vi "Initialize Waveforms V3.vi"(0 "Image Acquisition Parameters":T2={"Scan Type"=enum."Sample Scanning", "Scan Mode"=enum."XY", "Fast Axis Frequency (Hz)"=100.0, "Image Format"=128, "Line Accumulations"=1, "Frames Per Capture"=1, "Frames Accumulations"=1, "Image Dimension (um)"=[], "Number of Z Steps"=1, "Z Steps Size (um)"=1.0, "Pixel Size (nm)"=[]} {"Z Steps Size (um)" min=0.0; "Number of Z Steps" min=1; "Frames Accumulations" min=1; "Frames Per Capture" min=1; "Line Accumulations" min=1; "Image Format" items=["64 x 64"=64, "128 x 128"=128, "256 x 256"=256, "512 x 512"=512, "1024 x 1024"=1024, "2048 x 2048"=2048]}, 11 "Galvo Scale Factor":dbl=0.5 format="%#_13g") -> (4 "Waveform Data":T1)   [LabVIEW 2016]
uses:
  Type Defs/Image Acquisition Parameters.ctl
  Waveform Data.ctl
panel:
  in  "Waveform Data":T1
  out "Fast":cluster{dbl[], dbl[]}(graph)
  in  "Number Data of Points":i32=5000
  out "np":i32=5520
  out "total # lines":i32=296
  out "Slow":cluster{"t":dbl[], "L":dbl[]}(graph)
  out "% active scan":dbl=92.7536231884058
  out "dt":dbl=6.169792694965449e-06
  out "slow freq (Hz)":dbl=29.36231884057971
  out "T":dbl=0.03405725567620928
  out "t0":dbl=0.032823297137216184
  out "max dh/dt (V/s)":dbl=-1980.1192841578468
  out "constraint":dbl=7537.739130434783
  out "dh":dbl=0.07812500000000001
  out "k":dbl=7463.978793397228
  out "delta t (s)":dbl=0.0024679170779861796
  out "scan slope":dbl=31.656250000000004
  out "t image (s)":dbl=0.0315893385982231
  out "# lines flyback":i16=40
  in  "beta":dbl=0.0001 format="%0.2p"
  # "Copyright (C) 2010 Travis Gould\nCopyright (C) 2020 Edward S Allgeyer\n\nRedistribution and use in source and binary forms, with or without\nmodification, are permitted provided that the following conditions\nare met:\n\n1. Redistributions of source code must retain the above copyright\n   notice, this list of conditions and the following disclaimer.\n\n2. Redistributions in binary form must reproduce the above copyright\n   notice, this list of conditions and the following disclaimer in\n   the documentation and/or other materials provided with the\n   distribution.\n\n3. Neither the name of the copyright holder nor the names of its\n   contributors may be used to endorse or promote products derived\n   from this software without specific prior written permission.\n\nTHIS SOFTWARE IS PROVIDED BY THE COPYRIGHT HOLDERS AND CONTRIBUTORS\n\"AS IS\" AND ANY EXPRESS OR IMPLIED WARRANTIES, INCLUDING, BUT NOT\nLIMITED TO, THE IMPLIED WARRANTIES OF MERCHANTABILITY AND FITNESS\nFOR A PARTICULAR PURPOSE ARE DISCLAIMED. IN NO EVENT SHALL THE\nCOPYRIGHT HOLDER OR CONTRIBUTORS BE LIABLE FOR ANY DIRECT, INDIRECT,\nINCIDENTAL, SPECIAL, EXEMPLARY, OR CONSEQUENTIAL DAMAGES (INCLUDING,\nBUT NOT LIMITED TO, PROCUREMENT OF SUBSTITUTE GOODS OR SERVICES;\nLOSS OF USE, DATA, OR PROFITS; OR BUSINESS INTERRUPTION) HOWEVER\nCAUSED AND ON ANY THEORY OF LIABILITY, WHETHER IN CONTRACT, STRICT\nLIABILITY, OR TORT (INCLUDING NEGLIGENCE OR OTHERWISE) ARISING IN\nANY WAY OUT OF THE USE OF THIS SOFTWARE, EVEN IF ADVISED OF THE\nPOSSIBILITY OF SUCH DAMAGE."
  # "XY"
  # "Z"
  # "Length"
  # "Height"
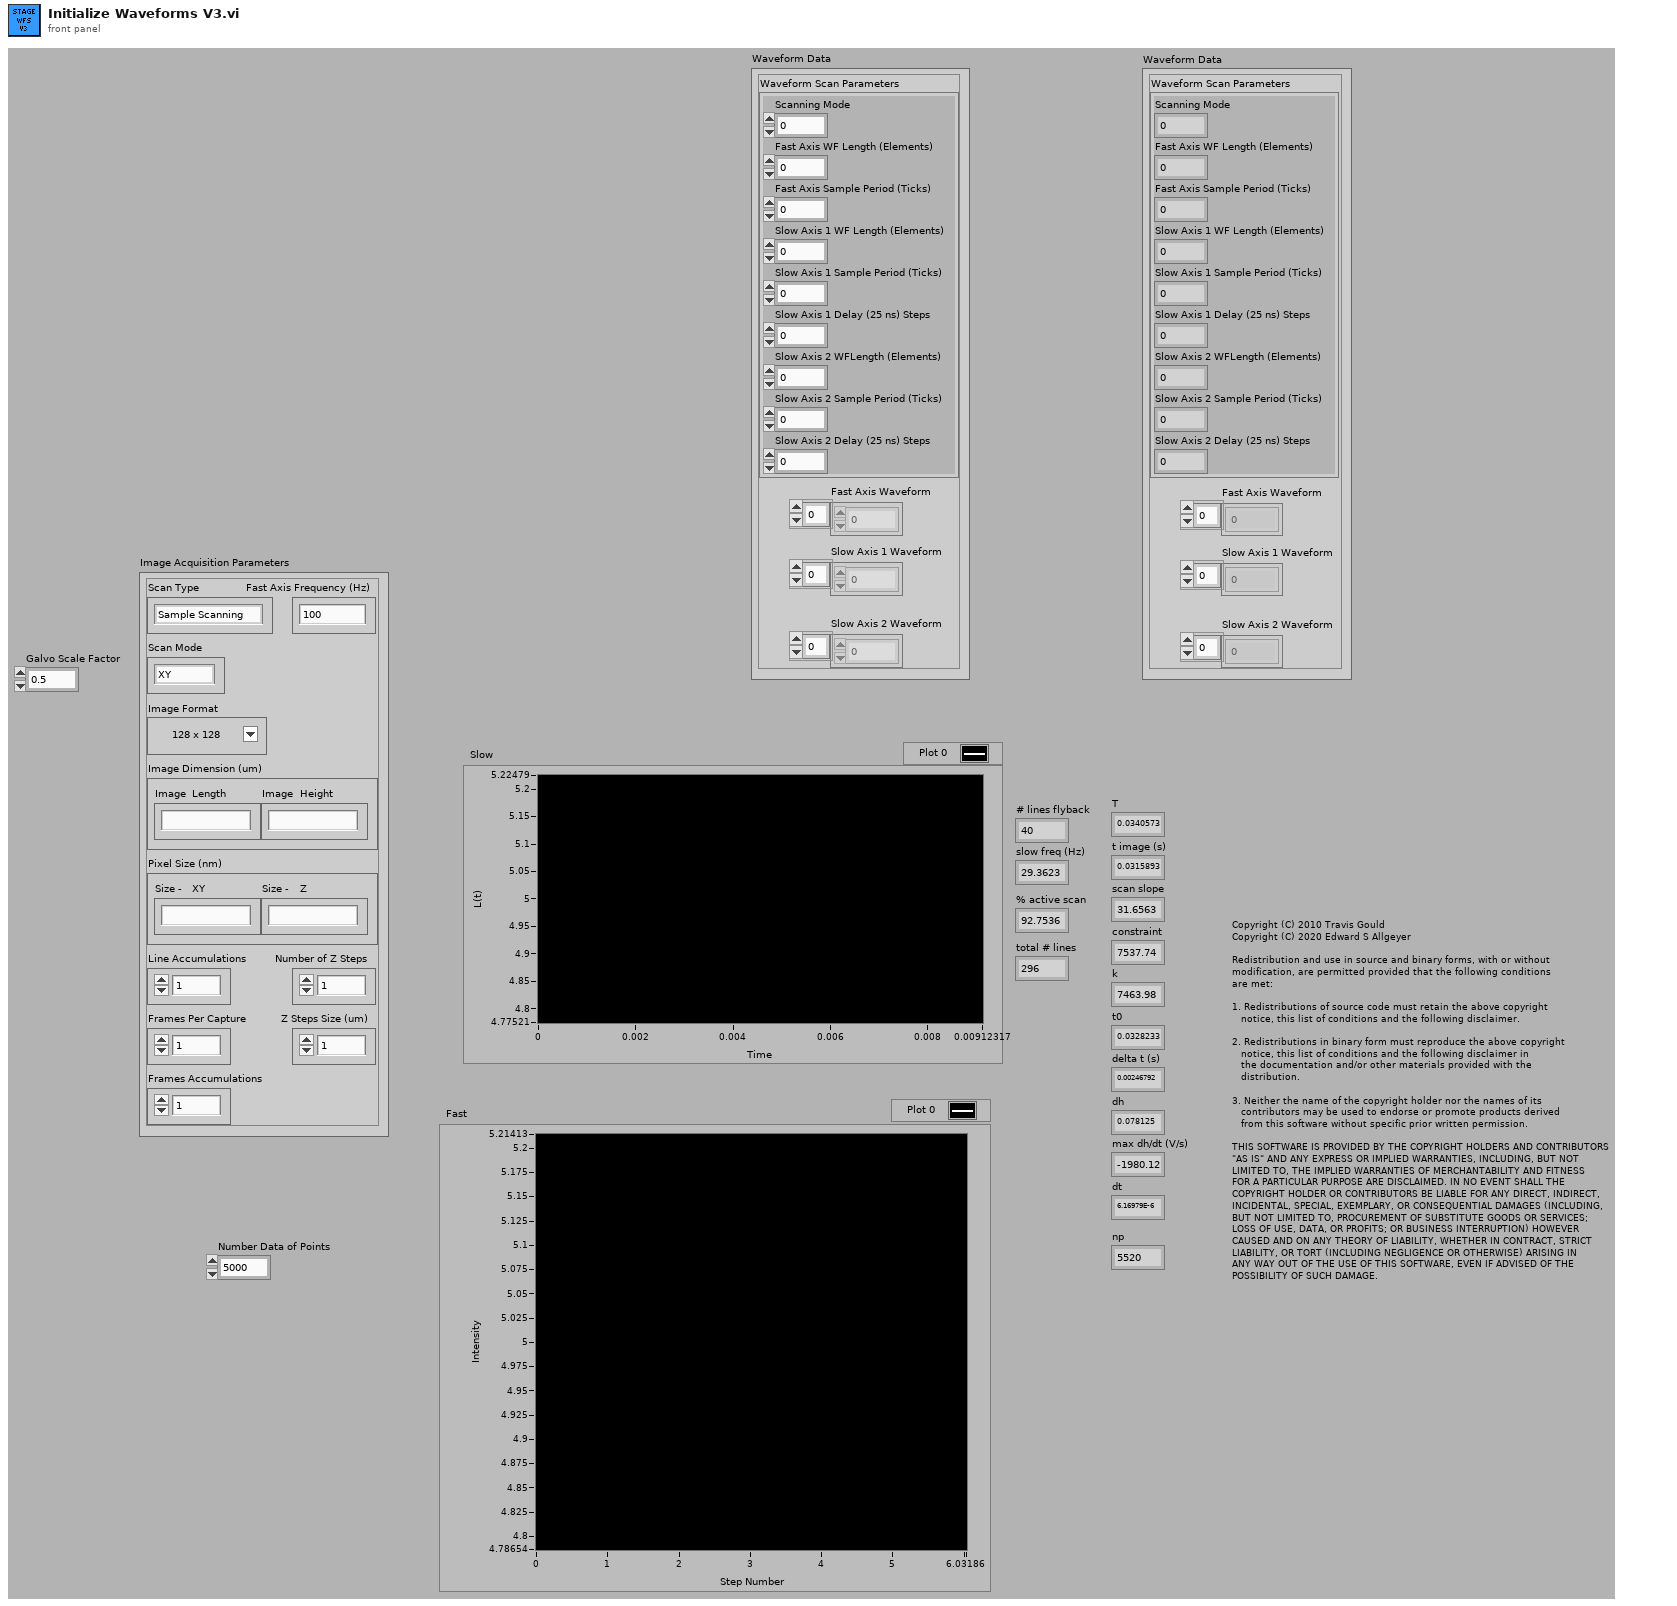
[diagram p1: front panel]
types:
  T1 = typedef "Waveform Data.ctl" = cluster{"Waveform Scan Parameters":cluster{"Scanning Mode":u8, "Fast Axis WF Length (Elements)":i32, "Fast Axis Sample Period (Ticks)":u32, "Slow Axis 1 WF Length (Elements)":i32, "Slow Axis 1 Sample Period (Ticks)":u32, "Slow Axis 1 Delay (25 ns) Steps":i32, "Slow Axis 2 WFLength (Elements)":i32, "Slow Axis 2 Sample Period (Ticks)":u32, "Slow Axis 2 Delay (25 ns) Steps":i32}, "Fast Axis Waveform":dbl[], "Slow Axis 1 Waveform":dbl[], "Slow Axis 2 Waveform":dbl[]}
  T2 = typedef "Image Acquisition Parameters.ctl" = cluster{"Scan Type":enum16{"Sample Scanning", "Beam Scanning"}, "Scan Mode":enum16{"XY", "XZ", "YZ", "XYZ"}, "Fast Axis Frequency (Hz)":dbl, "Image Format":u16, "Line Accumulations":u16, "Frames Per Capture":u16, "Frames Accumulations":u16, "Image Dimension (um)":dbl[], "Number of Z Steps":u8, "Z Steps Size (um)":dbl, "Pixel Size (nm)":dbl[]}
  T3 = cluster{"Scanning Mode":u8, "Fast Axis WF Length (Elements)":i32, "Fast Axis Sample Period (Ticks)":u32, "Slow Axis 1 WF Length (Elements)":i32, "Slow Axis 1 Sample Period (Ticks)":u32, "Slow Axis 1 Delay (25 ns) Steps":i32, "Slow Axis 2 WFLength (Elements)":i32, "Slow Axis 2 Sample Period (Ticks)":u32, "Slow Axis 2 Delay (25 ns) Steps":i32}
  T4 = typedef "Scan Parameters.ctl" = cluster{"Fast_Ax_Amp_V":dbl, "Fast_Ax_Off_V":dbl, "Slow_Ax_Amp_V":dbl, "Slow_Ax_Off_V ":dbl, "Slow_Ax_Max_V_VperS":dbl, "Slow_Ax1_Del25ns":i32, "Slow_Ax2_Del25ns":i32, "Stage_X_Off_V":dbl, "Stage_Y_Off_V":dbl, "Stage_Z_Off_V":dbl, "Galvo1_Off_V":dbl, "Galvo2_Off_V":dbl, "Last_Scan_Mode":enum16{"XY", "XZ", "YZ", "XYZ"}, "Current_Scan_Mode":enum16{"XY", "XZ", "YZ", "XYZ"}, "Fly_Back_Lines":u16, "Linear_Ramp_End":u32, "Z_Step_I16":i16, "Z_Start_I16":i16, "Laser_States _U32":u32, "590_Voltage_I16":i16, "775_AOM_Volt_I16":i16, "Blanking OFF":bool, "Unused_Axis_I16":i16}
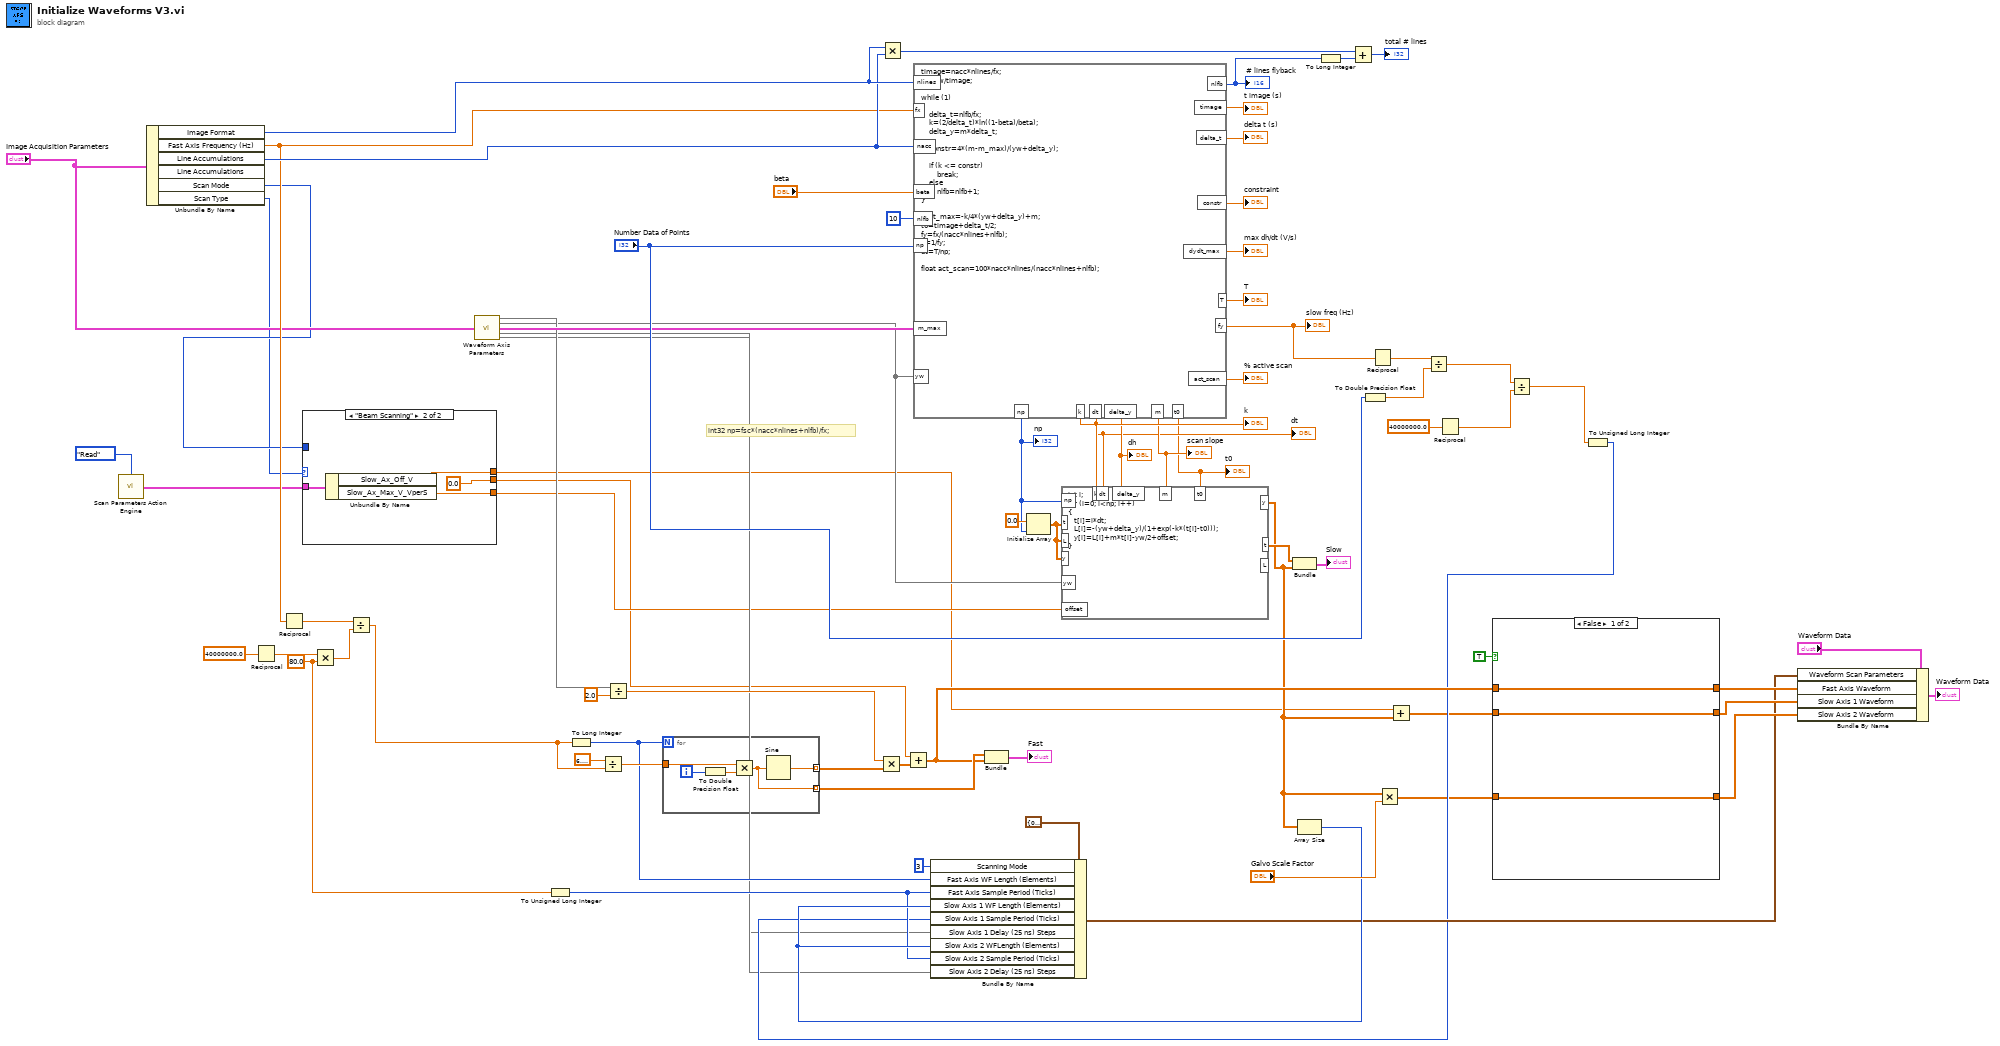
[diagram p0: block diagram]
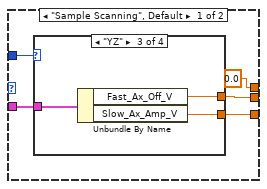
[diagram p2: hidden frame]
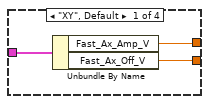
[diagram p3: hidden frame]
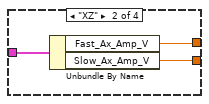
[diagram p4: hidden frame]
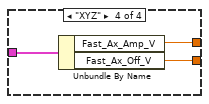
[diagram p5: hidden frame]
diagram:
  w33 = 80.0 ("y")
  # "int32 np=fsc*(nacc*nlines+nlfb)/fx;"
  n1 = call "Scan Parameters Action Engine.vi"("Action"=enum16{"Read", "Write"}."Read") -> ("Scan Parameters OUT"=w9:T4)  [unwired: 14 in]
  n2 = Unbundle By Name("Image Acquisition Parameters") -> ("Image Format"=w56:u16, "Fast Axis Frequency (Hz)"=w45:dbl, "Line Accumulations"=w55:u16, "Scan Mode"=w11:enum16{"XY", "XZ", "YZ", "XYZ"}, "Scan Type"=w7:enum16{"Sample Scanning", "Beam Scanning"})  [unwired: 1 out]
  n3 = Reciprocal(x=40000000.0) -> (1/x=w46:dbl)
  n4 = Reciprocal(x=w45) -> (1/x=w44:dbl)
  n5 = case shown="\"Beam Scanning\"" w7 {
    tunnel: w11 -> [w83 _]
    tunnel: w9 -> [w82 w99]
    tunnel: [w81 w98] -> w8
    tunnel: [w80 0.0 ("Galvo 2 Offset (V)")] -> w2
    tunnel: [0.0 ("Galvo 1 Offset (V)") w97] -> w4
    frame "Sample Scanning", Default {
      n6 = case shown="\"YZ\"" w83 {
        tunnel: w82 -> [w86 w89 w92 w95]
        tunnel: [w85 w88 w91 w94] -> w80
        tunnel: [w84 w87 w90 w93] -> w81
        frame "XY", Default {
          n7 = Unbundle By Name(w86) -> ("Fast_Ax_Amp_V"=w85:dbl, "Fast_Ax_Off_V"=w84:dbl)
        }
        frame "XZ" {
          n8 = Unbundle By Name(w89) -> ("Fast_Ax_Amp_V"=w88:dbl, "Slow_Ax_Amp_V"=w87:dbl)
        }
        frame "YZ" {
          n9 = Unbundle By Name(w92) -> ("Fast_Ax_Off_V"=w91:dbl, "Slow_Ax_Amp_V"=w90:dbl)
        }
        frame "XYZ" {
          n10 = Unbundle By Name(w95) -> ("Fast_Ax_Amp_V"=w94:dbl, "Fast_Ax_Off_V"=w93:dbl)
        }
      }
    }
    frame "Beam Scanning" {
      n11 = Unbundle By Name(w99) -> ("Slow_Ax_Off_V"=w97:dbl, "Slow_Ax_Max_V_VperS"=w98:dbl)
    }
  }
  n12 = Multiply(x=w46, y=w33) -> (x*y=w43:dbl)
  n13 = Divide(x=w44, y=w43) -> (x/y=w34:dbl)
  n14 = call "Waveform Axis Parameters.vi"("Image Acquisition Parameters"="Image Acquisition Parameters") -> (4:w16, 6:w15, "Scan Parameters"=w17:T4, 10:w13, 15:w14)  [unwired: 10 in]
  n15 = To Unsigned Long Integer(number=w33) -> (unsigned 32bit integer=w31:u32)
  n16 = To Long Integer(number=w34) -> (32bit integer=w35:i32)
  n17 = Divide(x=6.283185307179586, y=w34) -> (x/y=w53:dbl)
  n18 = Divide(x=w16, y=2.0) -> (x/y=w27:dbl)
  n19 = for {
    N: w35 -> [_]
    tunnel: w53 -> [w104]
    tunnel: [w101] -> w51 mode=indexing
    tunnel: [w102] -> w52 mode=indexing
    i -> [w100]
    n20 = To Double Precision Float(number=w100) -> (double precision float=w103:dbl)
    n21 = Multiply(x=w104, y=w103) -> (x*y=w102:dbl)
    n22 = Sine(x=w102) -> (sin(x)=w101:dbl)
  }
  n23 = Multiply(x=w27, y=w51) -> (x*y=w50:dbl[])
  n24 = Multiply(x=w56, y=w55) -> (x*y=w57:u16)
  n25 = Add(x=w2, y=w50) -> (x+y=w48:dbl[])
  n26 = formula code="timage=nacc*nlines/fx;\nm=yw/timage; \n\nwhile (1)\n{\n    delta_t=nlfb/fx;\n    k=(2/delta_t)*ln((1-beta)/beta);\n    delta_y=m*delta_t;\n    \n    constr=4*(m-m_max)/(yw+delta_y);\n\n    if (k <= constr)\n        break;\n    else\n        nlfb=nlfb+1;\n}\n\ndydt_max=-k/4*(yw+delta_y)+m;\nt0=timage+delta_t/2;\nfy=fx/(nacc*nlines+nlfb);\nT=1/fy;\ndt=T/np;\n\nfloat act_scan=100*nacc*nlines/(nacc*nlines+nlfb);"("yw"=w15, "fx"=w45, "nlines"=w56, "m_max"=w17, "beta"="beta", "nlfb"=i16 10 ("input variable"), "nacc"=w55, "np"="Number Data of Points") -> ("k"=w68:dbl, "delta_t"=→"delta t (s)":dbl, "timage"=→"t image (s)":dbl, "m"=w66:dbl, "delta_y"=w67:dbl, "constr"=→"constraint":dbl, "nlfb"=w60:i16, "dydt_max"=→"max dh/dt (V/s)":dbl, "t0"=w61:dbl, "T"=→"T":dbl, "fy"=w26:dbl, "dt"=w65:dbl, "act_scan"=→"% active scan":dbl, "np"=w69:i32)
  "# lines flyback" <- w60
  "scan slope" <- w66
  "k" <- w68
  "dh" <- w67
  "t0" <- w61
  "slow freq (Hz)" <- w26
  "dt" <- w65
  "np" <- w69
  n27 = Bundle(w52, w48) -> (→"Fast":cluster{dbl[], dbl[]})  [unwired: 1 in]
  n28 = Initialize Array(0.0 ("element"), w69) -> (w70:dbl[])
  n29 = formula code="int i;\nfor (i=0; i<np; i++)\n{\n   t[i]=i*dt;\n   L[i]=-(yw+delta_y)/(1+exp(-k*(t[i]-t0)));\n   y[i]=L[i]+m*t[i]-yw/2+offset;\n}"("np"=w69, "t"=w70, "L"=w70, "y"=w70, "offset"=w8, "k"=w68, "dt"=w65, "yw"=w15, "delta_y"=w67, "m"=w66, "t0"=w61) -> ("t"=w64:dbl[], "y"=w6:dbl[])  [unwired: 1 out]
  n30 = Bundle("t"=w64, "y"=w6) -> (→"Slow":cluster{"t":dbl[], "y":dbl[]})  [unwired: 1 out]
  n31 = Array Size(array=w6) -> (size(s)=w32:i32)
  n32 = To Long Integer(number=w60) -> (32bit integer=w58:i32)
  n33 = Add(x=w57, y=w58) -> (x+y=→"total # lines":i32)
  n34 = To Double Precision Float(number="Number Data of Points") -> (double precision float=w24:dbl)
  n35 = Reciprocal(x=w26) -> (1/x=w25:dbl)
  n36 = Multiply(x=w6, y="Galvo Scale Factor") -> (x*y=w3:dbl[])
  n37 = Add(x=w4, y=w6) -> (x+y=w5:dbl[])
  n38 = Divide(x=w25, y=w24) -> (x/y=w21:dbl)
  n39 = Reciprocal(x=40000000.0) -> (1/x=w20:dbl)
  n40 = case shown="False" TRUE {
    tunnel: w5 -> [w106 w109]
    tunnel: w48 -> [w107 w110]
    tunnel: w3 -> [w105 w108]
    tunnel: [w107 w110] -> w40
    tunnel: [w106 w109] -> w39
    tunnel: [w105 w108] -> w38
    frame False {
    }
    frame True {
    }
  }
  n41 = Divide(x=w21, y=w20) -> (x/y=w19:dbl)
  n42 = To Unsigned Long Integer(number=w19) -> (unsigned 32bit integer=w18:u32)
  n43 = Bundle By Name(cluster=T3 {"Scanning Mode"=0, "Fast Axis WF Length (Elements)"=0, "Fast Axis Sample Period (Ticks)"=0, "Slow Axis 1 WF Length (Elements)"=0, "Slow Axis 1 Sample Period (Ticks)"=0, "Slow Axis 1 Delay (25 ns) Steps"=0, "Slow Axis 2 WFLength (Elements)"=0, "Slow Axis 2 Sample Period (Ticks)"=0, "Slow Axis 2 Delay (25 ns) Steps"=0} ("Waveform Scan Parameters"), "Scanning Mode"=u8 3, "Fast Axis WF Length (Elements)"=w35, "Fast Axis Sample Period (Ticks)"=w31, "Slow Axis 1 WF Length (Elements)"=w32, "Slow Axis 1 Sample Period (Ticks)"=w18, "Slow Axis 1 Delay (25 ns) Steps"=w13, "Slow Axis 2 WFLength (Elements)"=w32, "Slow Axis 2 Sample Period (Ticks)"=w31, "Slow Axis 2 Delay (25 ns) Steps"=w14) -> (w30:T3)
  n44 = Bundle By Name(cluster="Waveform Data", "Waveform Scan Parameters"=w30, "Fast Axis Waveform"=w40, "Slow Axis 1 Waveform"=w39, "Slow Axis 2 Waveform"=w38) -> (→"Waveform Data":T1)
